vi "FixBadRect.vi"(0 "Rectangle In":T1) -> (1 "Fixed?":bool=TRUE, 2 "Rectangle Out":T1)   [LabVIEW 2015]
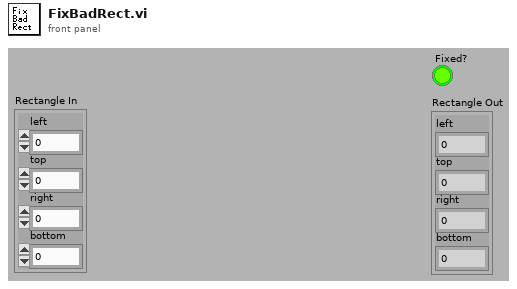
[diagram p1: front panel]
types:
  T1 = cluster{"left":i16, "top":i16, "right":i16, "bottom":i16}
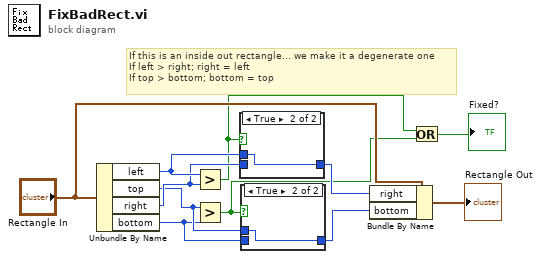
[diagram p0: block diagram]
diagram:
  # "If this is an inside out rectangle... we make it a degenerate one\nIf left > right; right = left\nIf top > bottom; bottom = top"
  n1 = Unbundle By Name("Rectangle In") -> ("left"=w11:i16, "top"=w9:i16, "right"=w10:i16, "bottom"=w8:i16)
  n2 = Greater?(x=w11, y=w10) -> (0:w2:bool)
  n3 = Greater?(x=w9, y=w8) -> (0:w1:bool)
  n4 = case shown="True" w2 {
    tunnel: w11 -> [_ w13]
    tunnel: w10 -> [w12 _]
    tunnel: [w12 w13] -> w5
    frame False {
    }
    frame True {
    }
  }
  n5 = case shown="True" w1 {
    tunnel: w9 -> [_ w15]
    tunnel: w8 -> [w14 _]
    tunnel: [w14 w15] -> w4
    frame False {
    }
    frame True {
    }
  }
  n6 = Bundle By Name(cluster="Rectangle In", "right"=w5, "bottom"=w4) -> (→"Rectangle Out":T1)
  n7 = Or(x=w2, y=w1) -> (x .or. y?=→"Fixed?":bool)
